vi "mxwScript_API_SetVal_CodeGenRecipe.vi"(7 "itemSelectType":T1, 8 "error in (no error)":errorcluster, 9 "codeGenRecipe":T3, 10 "label":string, 11 "index":i32) -> (0 "error out":errorcluster, 3 "parameter":T2)   [LabVIEW 2017]
uses:
  codeGenAPISupport.llb/cgAPI_mxwScript_Parameter.ctl
  codeGenAPISupport.llb/cgAPI_mxwScript_SetParm_ItemSelectType.ctl
  codeGenAPISupport.llb/cgAPI_mxwCodeGenCompleteRecipe.ctl
  codeGenAPISupport.llb/cgAPI_mxwScript_TemplateInfo.ctl
  codeGenAPISupport.llb/cgAPI_mxwScript_Wire_InputWireConnection.ctl
  codeGenAPISupport.llb/cgAPI_mxwScript_ConnPaneConnectionSpec.ctl
  codeGenAPISupport.llb/cgAPI_mxwScript_OptionData.ctl
  codeGenAPISupport.llb/cgAPI_mxwScript_SetParm_CodeGenRecipeN.ctl
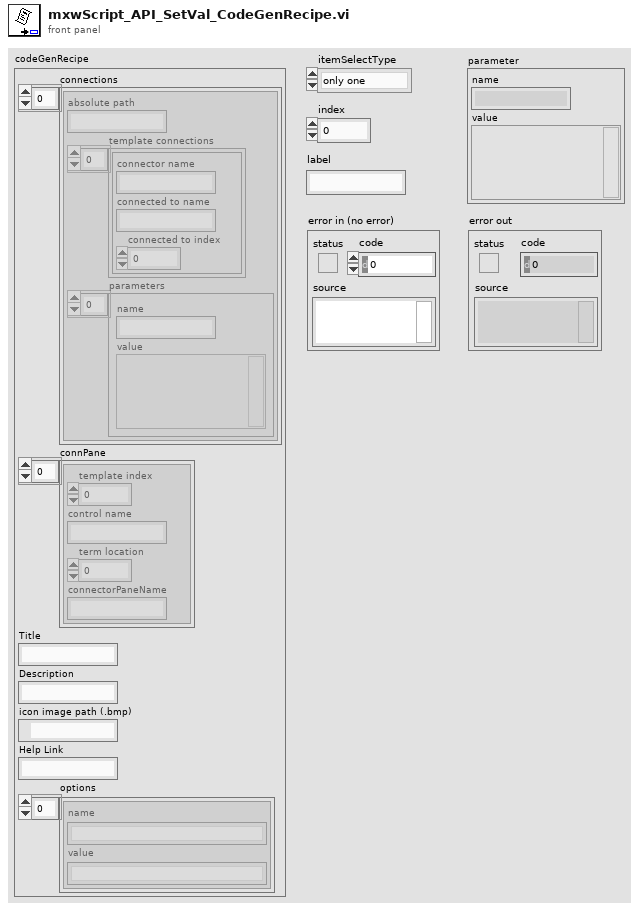
[diagram p1: front panel]
types:
  T1 = typedef "cgAPI_mxwScript_SetParm_ItemSelectType.ctl" = enum16{"only one", "index", "label", "VI name", "legacy"}
  T2 = typedef "cgAPI_mxwScript_Parameter.ctl" = cluster{"name":string, "value":variant}
  T3 = typedef "cgAPI_mxwCodeGenCompleteRecipe.ctl" = cluster{"connections":T4[], "connPane":T6[], "Title":string, "Description":string, "icon image path (.bmp)":path, "Help Link":string, "options":T7[]}
  T4 = typedef "cgAPI_mxwScript_TemplateInfo.ctl" = cluster{"absolute path":string, "template connections":T5[], "parameters":T2[]}
  T5 = typedef "cgAPI_mxwScript_Wire_InputWireConnection.ctl" = cluster{"connector name":string, "connected to name":string, "connected to index":i32}
  T6 = typedef "cgAPI_mxwScript_ConnPaneConnectionSpec.ctl" = cluster{"template index":u32, "control name":string, "term location":i32, "connectorPaneName":string}
  T7 = typedef "cgAPI_mxwScript_OptionData.ctl" = cluster{"name":string, "value":string}
  T8 = typedef "cgAPI_mxwScript_SetParm_CodeGenRecipeN.ctl" = cluster{"itemSelectType":T1, "index":i32, "label":string, "CodeGenRecipe":T3}
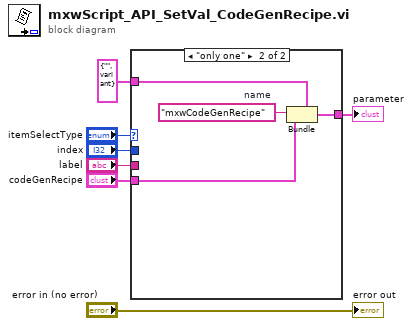
[diagram p0: block diagram]
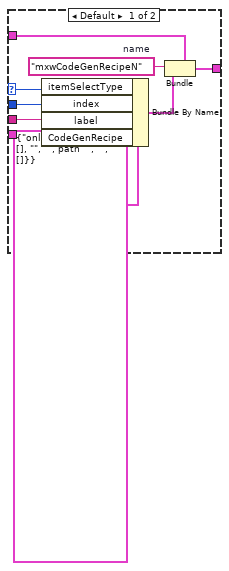
[diagram p2: hidden frame]
diagram:
  n1 = case shown="\"only one\"" "itemSelectType" {
    selector: "itemSelectType" -> [w13 _]
    tunnel: "index" -> [w16 _]
    tunnel: "label" -> [w15 _]
    tunnel: "codeGenRecipe" -> [w14 w17]
    tunnel: T2 {"name"="", "value"=variant} ("parameter") -> [w11 w19]
    tunnel: [w9 w18] -> w1
    frame Default {
      w12 = "mxwCodeGenRecipeN"  # name
      n2 = Bundle By Name(cluster=T8 {"itemSelectType"=enum."only one", "index"=0, "label"="", "CodeGenRecipe"={"connections"=[], "connPane"=[], "Title"="", "Description"="", "icon image path (.bmp)"=path "", "Help Link"="", "options"=[]}} ("codeGenRecipeN"), "itemSelectType"=w13, "index"=w16, "label"=w15, "CodeGenRecipe"=w14) -> (w10:T8)
      n3 = Bundle(cluster=w11, "name"=w12, "value"=w10) -> (w9:T2)
    }
    frame "only one" {
      w20 = "mxwCodeGenRecipe"  # name
      n4 = Bundle(cluster=w19, "name"=w20, "value"=w17) -> (w18:T2)
    }
  }
  "parameter" <- w1
  "error out" <- "error in (no error)"
